vi "Read Binary Configuration.vi"(7 "Type":T1, 8 "error in (no error)":errorcluster, 9 "Default If Not Found":variant, 10 "Name":string, 11 "IConfiguration in":refnum<class "IConfiguration.lvclass">) -> (0 "error out":errorcluster, 1 "Not Found?":bool, 2 "Value":variant, 3 "IConfiguration out":refnum<class "IConfiguration.lvclass">)   [LabVIEW 2020, in "Configuration.lvlib" / "IConfiguration.lvclass"]
uses:
  <vilib>/gpm_packages/@cs/Configuration/Source/IConfiguration/IConfiguration.lvclass
  <vilib>/Utility/Data Type/Type Definitions/Data Type.ctl
  <vilib>/Utility/error.llb/Error Cluster From Error Code.vi
  <vilib>/ErrorRing/Error Ring.xnode
  <vilib>/Utility/Data Type/NI_Data Type.lvlib
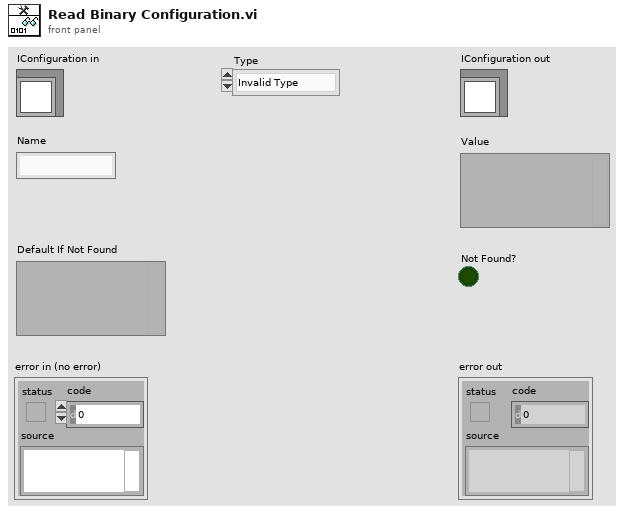
[diagram p1: front panel]
types:
  T1 = typedef "NI_Data Type.lvlib/Data Type.ctl" = enum8{"Invalid Type", "Void", "I8", "I16", "I32", "I64", "U8", "U16", "U32", "U64", "Single Float", "Double Float", "Extended Float", "Single Complex", "Double Complex", "Extended Complex", "Enum U8", "Enum U16", "Enum U32", "Enum U64", "Single Float With Unit", "Double Float With Unit", "Extended Float With Unit", "Single Complex with Unit", "Double Complex with Unit", "Extended Complex with Unit", "Boolean", "String", "Path", "Picture", "Tag", "Array", "Cluster", "Variant", "LV Variant", "Waveform", "Timestamp", "Digital Waveform", "Digital Data", "ExpressData", "Refnum", "External Data", "VI", "Poly VI", "LabVIEW Class Instance", "Fixed Point", "Set Collection", "Map Collection"}
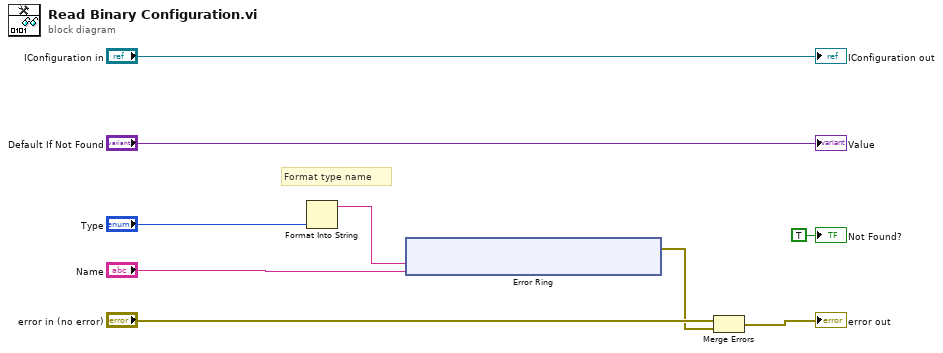
[diagram p0: block diagram]
diagram:
  # "Format type name"
  n1 = Format Into String("Type") -> (resulting string=w6:string)  [unwired: 3 in, 1 out]
  n2 = xnode "Error Ring"("parameter 0"=w6, "parameter 1"="Name") -> ("error out"=w2:errorcluster)
  n3 = Merge Errors("error in (no error)", w2) -> (→"error out":errorcluster)
  "IConfiguration out" <- "IConfiguration in"
  "Value" <- "Default If Not Found"
  "Not Found?" <- TRUE ("Not Found?")
